vi "CheckFreq.vi"(0 "Motor in":refnum<class "Motor.lvclass">, 5 "Current Frequency":dbl, 7 "Center Frequency(GHz)":dbl=140.18, 9 "Range(GHz)":dbl, 11 "error in (no error)":errorcluster) -> (4 "Motor out":refnum<class "Motor.lvclass">, 6 "Freq_in Range":bool, 15 "error out":errorcluster)   [LabVIEW 2019, in "Motor.lvclass"]
uses:
  Motor.lvclass
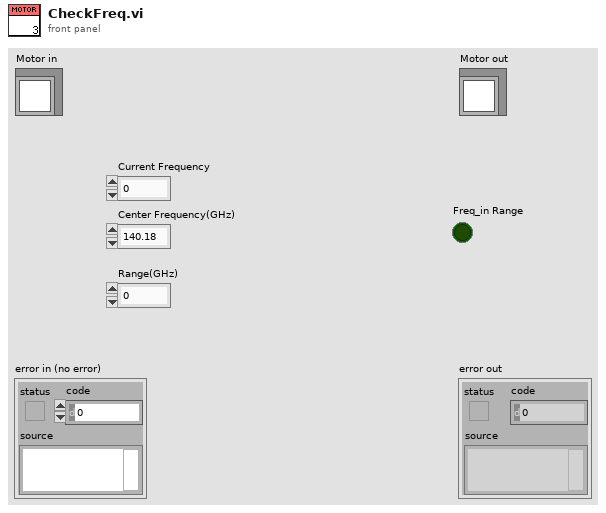
[diagram p1: front panel]
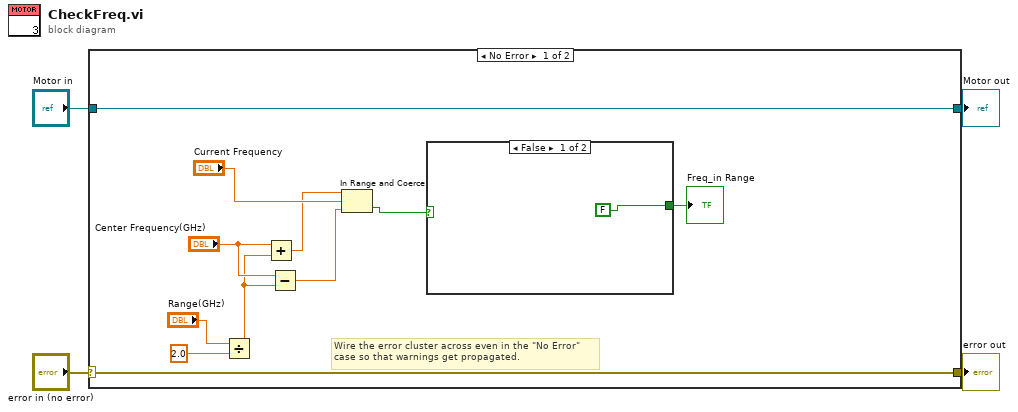
[diagram p0: block diagram]
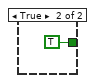
[diagram p2: hidden frame]
diagram:
  n1 = case shown="No Error" "error in (no error)" {
    selector: "error in (no error)" -> [w14 w19]
    tunnel: [w14 w19] -> w3
    tunnel: [w15 w18] -> w1
    tunnel: "Motor in" -> [w15 w18]
    frame No Error {
      # "Wire the error cluster across even in the \"No Error\"\ncase so that warnings get propagated."
      n2 = Divide(x="Range(GHz)", y=2.0) -> (x/y=w8:dbl)
      n3 = Add(x="Center Frequency(GHz)", y=w8) -> (x+y=w10:dbl)
      n4 = Subtract(x="Center Frequency(GHz)", y=w8) -> (x-y=w7:dbl)
      n5 = In Range and Coerce(upper limit=w10, x="Current Frequency", lower limit=w7) -> (In Range?=w6:bool)  [unwired: 1 out]
      n6 = case shown="False" w6 {
        tunnel: [FALSE ("Freq_in Range") TRUE ("Freq_in Range")] -> w5
        frame False {
        }
        frame True {
        }
      }
      "Freq_in Range" <- w5
    }
    frame Error {
    }
  }
  "error out" <- w3
  "Motor out" <- w1
